vi "Write Image delays.vi"(8 "error in (no error)":errorcluster, 10 "Image Delays":u64, 11 "Header in":refnum<class "Simulated_Header.lvclass">) -> (0 "error out":errorcluster, 3 "Header out":refnum<class "Simulated_Header.lvclass">)   [LabVIEW 2018, in "Simulated_Header.lvclass"]
uses:
  Simulated_Header.lvclass
  Simulated_Header.lvclass/Simulated_Header.ctl
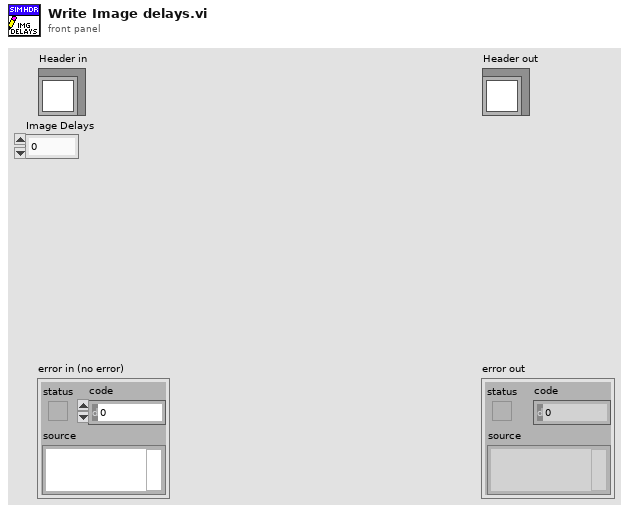
[diagram p1: front panel]
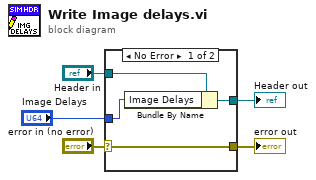
[diagram p0: block diagram]
diagram:
  n1 = case shown="No Error" "error in (no error)" {
    selector: "error in (no error)" -> [w9 w10]
    tunnel: [w9 w10] -> w4
    tunnel: [w7 w11] -> w2
    tunnel: "Header in" -> [w8 w11]
    tunnel: "Image Delays" -> [w6 _]
    frame No Error {
      n2 = Bundle By Name(cluster=w8, "Image Delays"=w6) -> (w7:refnum<class "Simulated_Header.lvclass">)
    }
    frame Error {
    }
  }
  "error out" <- w4
  "Header out" <- w2
